vi "RSNRPZ Set Scope Realtime State.vi"(8 "error in (no error)":errorcluster, 9 "Realtime (F: Off)":bool, 10 "Channel (1)":i32=1, 11 "VISA session":refnum<visa-resource-name> caption="VISA resource name") -> (0 "error out":errorcluster, 3 "dup VISA session":refnum<visa-resource-name> caption="VISA resource name")   [LabVIEW 2010]
doc: "In the default state (OFF), each measurement sequence from the sensor is averaged over several sequences. Since the measured values of a sequence may be closer to each other in time than the measurements, several measurement sequences with a slight time offset are also superimposed on the desired sequence. With the state turned ON - this effect can be switched off, which may increase the measurement speed. This ensures that the measured values of an individual sequence are immediately delivered.\n\nNote:\n\n1) This VI is not available for NRP-Z51.\n\nRemote-control command(s):\nSENS:TRAC:REAL ON | OFF"
uses:
  rsnrpz_32.dll
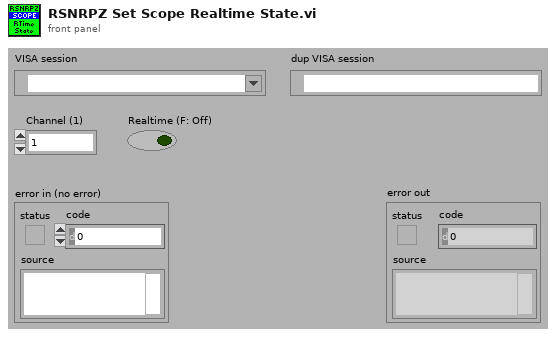
[diagram p1: front panel]
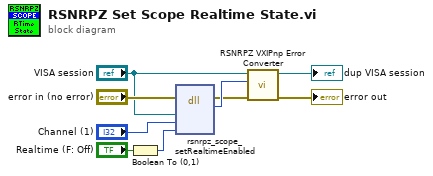
[diagram p0: block diagram]
diagram:
  n1 = Boolean To (0,1)(Boolean="Realtime (F: Off)") -> (0, 1=w6:i16)
  n2 = dll-call lib="rsnrpz_32.dll" fn="rsnrpz_scope_setRealtimeEnabled"(error in="error in (no error)", "VISA Session"="VISA session", "Channel"="Channel (1)", "Realtime"=w6) -> (error out=w5:errorcluster, "Status"=w8:i32)  [unwired: 5 in, 1 out]
  n3 = call <instrlib>:"RSNRPZ VXIPnp Error Converter.vi"("error in"=w5, "VXIPnp error code"=w8, "VISA session"="VISA session") -> ("error out"=→"error out":errorcluster, "dup VISA session"=→"dup VISA session":refnum<visa-resource-name>)  [unwired: 7 in]
